vi "万能日期时间字符串解析.vi"(6 "分隔符(空格)":string=" " caption="日期时间分隔符(空格)", 11 "日期时间字符串":string="2017/12.30 12-12_12") -> (3 "时间标识":timestamp, 4 "格式":enum16{"无意义", "日期时间", "仅日期", "仅时间"}(ring))   [LabVIEW 2017]
uses:
  <vilib>/Utility/miscctls.llb/LVDateTimeRec.ctl
panel:
  out "6":string
  out "5":string
  out "4":string
  out "3":string
  out "2":string
  out "1":string
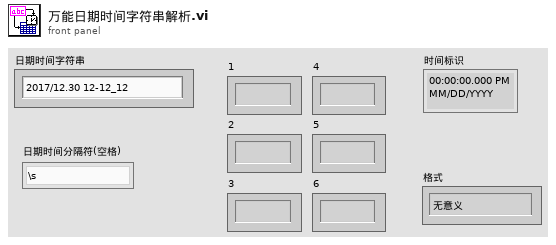
[diagram p1: front panel]
types:
  T1 = typedef "LVDateTimeRec.ctl" = cluster{"fractional second":dbl, "second":i32, "minute":i32, "hour":i32, "day of month":i32, "month":i32, "year":i32, "day of week":i32, "day of year":i32, "DST":i32}
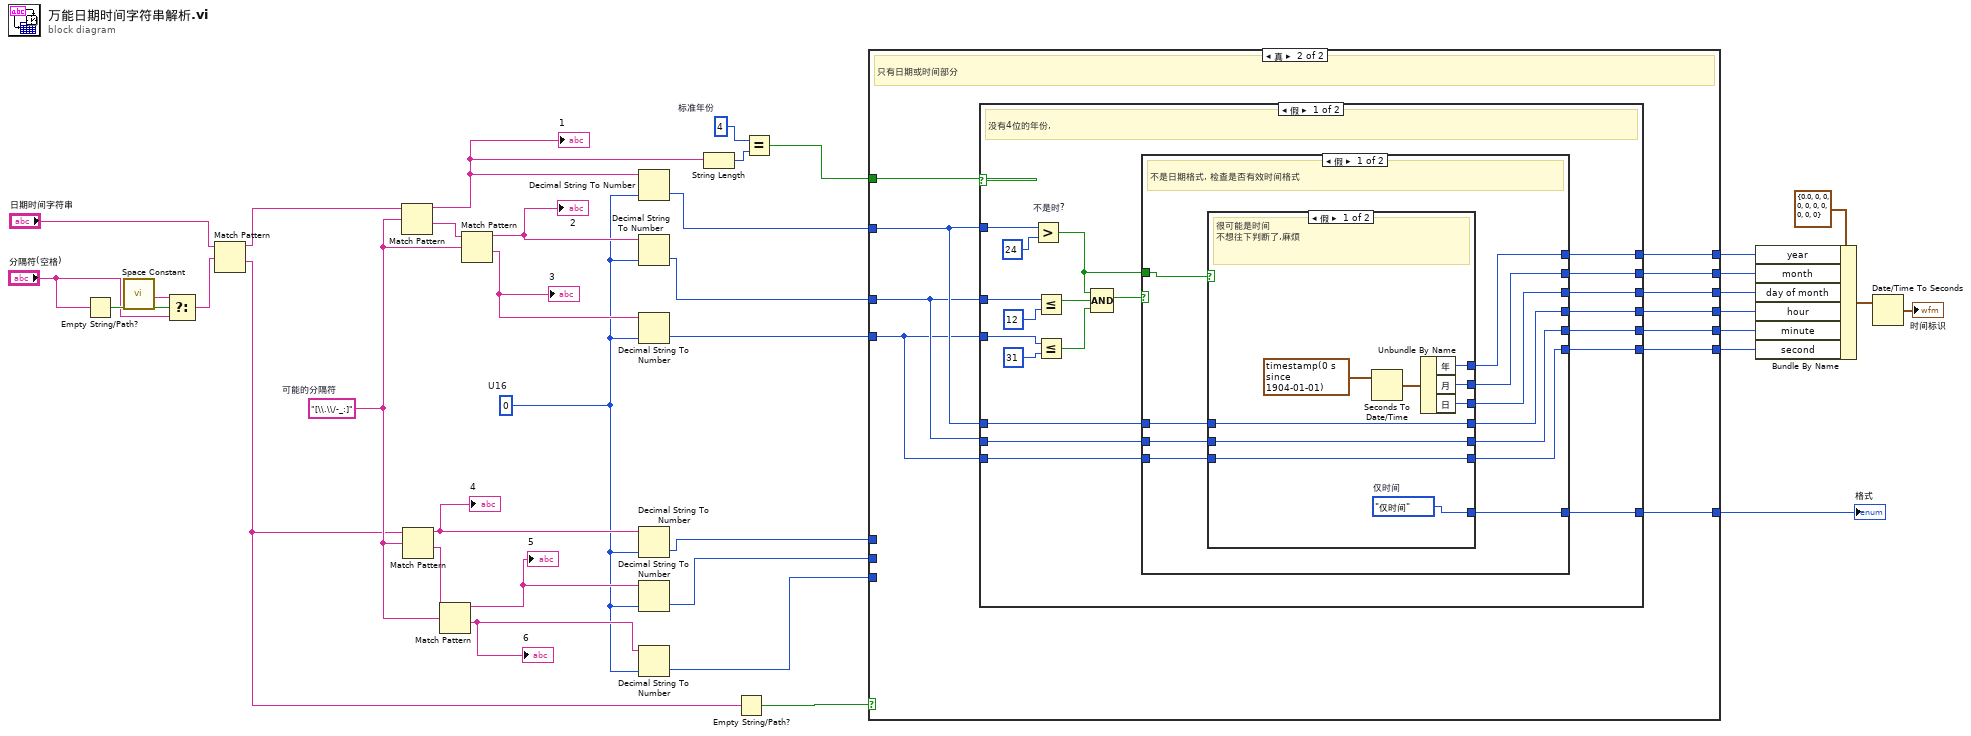
[diagram p0: block diagram]
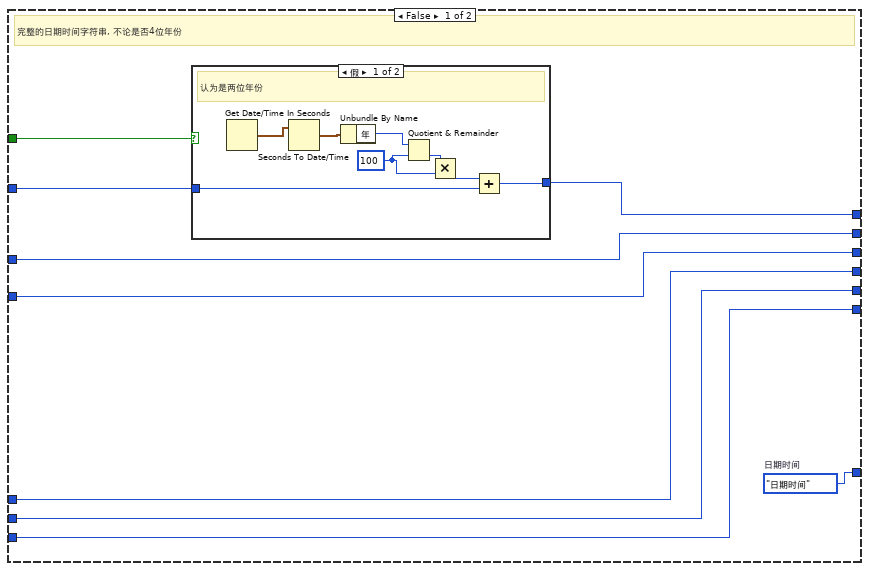
[diagram p2: hidden frame]
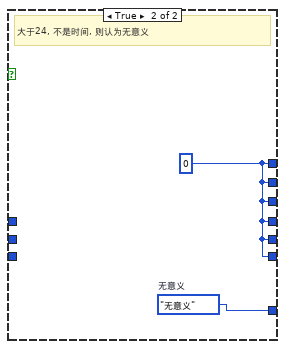
[diagram p4: hidden frame]
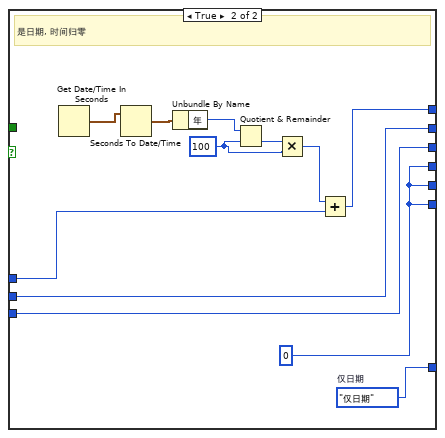
[diagram p5: hidden frame]
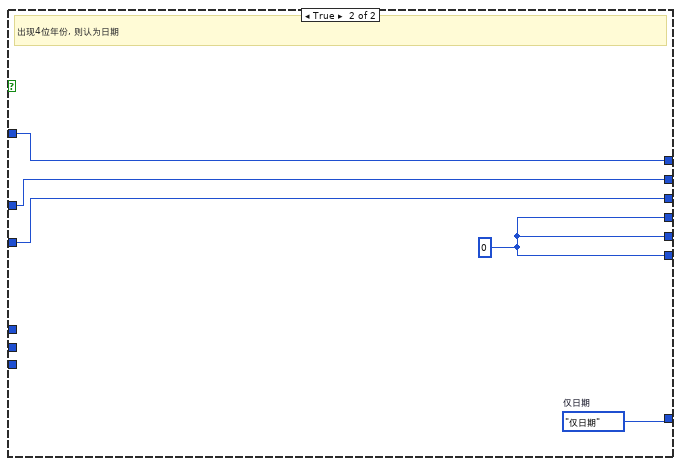
[diagram p6: hidden frame]
diagram:
  w22 = u16 0  # U16
  w24 = 4  # 标准年份
  w34 = "[\\.\\/-_:]"  # 可能的分隔符
  n1 = Empty String/Path?(string/path="分隔符(空格)") -> (empty?=w4:bool)
  n2 = call <vilib>:"Space Constant.vi"() -> ("String"=w3:string)
  n3 = Select(t=w3, s=w4, f="分隔符(空格)") -> (s? t:f=w1:string)
  n4 = Match Pattern(string="日期时间字符串", regular expression=w1) -> (before substring=w36:string, after substring=w27:string)  [unwired: 1 in, 2 out]
  n5 = Match Pattern(string=w36, regular expression=w34) -> (before substring=w26:string, after substring=w35:string)  [unwired: 1 in, 2 out]
  "1" <- w26
  n6 = Match Pattern(string=w27, regular expression=w34) -> (before substring=w30:string, after substring=w33:string)  [unwired: 1 in, 2 out]
  "4" <- w30
  n7 = Match Pattern(string=w33, regular expression=w34) -> (before substring=w29:string, after substring=w28:string)  [unwired: 1 in, 2 out]
  "5" <- w29
  "6" <- w28
  n8 = Match Pattern(string=w35, regular expression=w34) -> (before substring=w32:string, after substring=w31:string)  [unwired: 1 in, 2 out]
  "2" <- w32
  "3" <- w31
  n9 = Decimal String To Number(string=w26, default (0L)=w22) -> (number=w20:u16)  [unwired: 1 in, 1 out]
  n10 = Decimal String To Number(string=w32, default (0L)=w22) -> (number=w19:u16)  [unwired: 1 in, 1 out]
  n11 = Decimal String To Number(string=w31, default (0L)=w22) -> (number=w18:u16)  [unwired: 1 in, 1 out]
  n12 = Decimal String To Number(string=w30, default (0L)=w22) -> (number=w17:u16)  [unwired: 1 in, 1 out]
  n13 = Decimal String To Number(string=w29, default (0L)=w22) -> (number=w16:u16)  [unwired: 1 in, 1 out]
  n14 = Decimal String To Number(string=w28, default (0L)=w22) -> (number=w15:u16)  [unwired: 1 in, 1 out]
  n15 = String Length(string=w26) -> (length=w25:i32)
  n16 = Empty String/Path?(string/path=w27) -> (empty?=w23:bool)
  n17 = Equal?(x=w24, y=w25) -> (x = y?=w21:bool)
  n18 = case shown="真" w23 {
    tunnel: w21 -> [w46 w66]
    tunnel: w20 -> [w45 w59]
    tunnel: w19 -> [w43 w58]
    tunnel: w18 -> [w42 w57]
    tunnel: w17 -> [w41 _]
    tunnel: w16 -> [w40 _]
    tunnel: w15 -> [w39 _]
    tunnel: [w44 w65] -> w12
    tunnel: [w43 w64] -> w11
    tunnel: [w42 w63] -> w10
    tunnel: [w41 w62] -> w9
    tunnel: [w40 w61] -> w8
    tunnel: [w39 w60] -> w7
    tunnel: [w38 w56] -> w5
    frame False {
      w38 = enum16{"无意义", "日期时间", "仅日期", "仅时间"}."日期时间"  # 日期时间
      # "完整的日期时间字符串, 不论是否4位年份"
      n19 = case shown="假" w46 {
        tunnel: w45 -> [w50 w55]
        tunnel: [w49 w55] -> w44
        frame False {
          w47 = 100 ("y")
          # "认为是两位年份"
          n20 = Get Date/Time In Seconds() -> (seconds since 1Jan1904=w54:timestamp)
          n21 = Seconds To Date/Time(time stamp (now)=w54) -> (date time rec=w53:T1)  [unwired: 1 in]
          n22 = Unbundle By Name(w53) -> ("年"=w52:i32)
          n23 = Quotient & Remainder(x=w52, y=w47) -> (floor(x/y)=w51:i32)  [unwired: 1 out]
          n24 = Multiply(x=w51, y=w47) -> (x*y=w48:i32)
          n25 = Add(x=w48, y=w50) -> (x+y=w49:i32)
        }
        frame True {
          # "4位年份"
        }
      }
    }
    frame True {
      # "只有日期或时间部分"
      n26 = case shown="假" w66 {
        tunnel: w59 -> [w86 w125]
        tunnel: w58 -> [w84 w124]
        tunnel: w57 -> [w82 w123]
        tunnel: [w76 w125] -> w65
        tunnel: [w75 w124] -> w64
        tunnel: [w74 w123] -> w63
        tunnel: [w70 w122] -> w62
        tunnel: [w69 w122] -> w61
        tunnel: [w68 w122] -> w60
        tunnel: w59 -> [w73 _]
        tunnel: w58 -> [w72 _]
        tunnel: w57 -> [w71 _]
        tunnel: [w67 w121] -> w56
        frame False {
          # "没有4位的年份,"
          n27 = Greater? "不是时?"(x=w86, y=u16 24) -> (0:w77:bool)
          n28 = Less Or Equal?(x=w84, y=u16 12) -> (x <= y?=w79:bool)
          n29 = Less Or Equal?(x=w82, y=u16 31) -> (x <= y?=w78:bool)
          n30 = Compound Arithmetic op=AND ("复合运算")(w77, w79, w78) -> (w80:bool)
          n31 = case shown="假" w80 {
            tunnel: w77 -> [w97 _]
            tunnel: [w96 w112] -> w76
            tunnel: [w95 w120] -> w75
            tunnel: [w94 w119] -> w74
            tunnel: w73 -> [w93 w113]
            tunnel: w72 -> [w92 w120]
            tunnel: w71 -> [w91 w119]
            tunnel: [w90 w118] -> w70
            tunnel: [w89 w118] -> w69
            tunnel: [w88 w118] -> w68
            tunnel: [w87 w109] -> w67
            frame False {
              # "不是日期格式, 检查是否有效时间格式"
              n32 = case shown="假" w97 {
                tunnel: [w104 w108] -> w96
                tunnel: [w103 w108] -> w95
                tunnel: [w102 w108] -> w94
                tunnel: w93 -> [w101 _]
                tunnel: w92 -> [w100 _]
                tunnel: w91 -> [w99 _]
                tunnel: [w101 w108] -> w90
                tunnel: [w100 w108] -> w89
                tunnel: [w99 w108] -> w88
                tunnel: [w98 w107] -> w87
                frame False {
                  w98 = enum16{"无意义", "日期时间", "仅日期", "仅时间"}."仅时间"  # 仅时间
                  # "很可能是时间\n不想往下判断了,麻烦"
                  n33 = Seconds To Date/Time(time stamp (now)=timestamp(0 s since 1904-01-01) ("时间标识")) -> (date time rec=w106:T1)  [unwired: 1 in]
                  n34 = Unbundle By Name(w106) -> ("年"=w104:i32, "月"=w103:i32, "日"=w102:i32)
                }
                frame True {
                  w107 = enum16{"无意义", "日期时间", "仅日期", "仅时间"}."无意义"  # 无意义
                  w108 = 0 ("年")
                  # "大于24, 不是时间, 则认为无意义"
                }
              }
            }
            frame True {
              w109 = enum16{"无意义", "日期时间", "仅日期", "仅时间"}."仅日期"  # 仅日期
              w110 = 100 ("y")
              w118 = 0 ("年")
              # "是日期, 时间归零"
              n35 = Get Date/Time In Seconds() -> (seconds since 1Jan1904=w117:timestamp)
              n36 = Seconds To Date/Time(time stamp (now)=w117) -> (date time rec=w116:T1)  [unwired: 1 in]
              n37 = Unbundle By Name(w116) -> ("年"=w115:i32)
              n38 = Quotient & Remainder(x=w115, y=w110) -> (floor(x/y)=w114:i32)  [unwired: 1 out]
              n39 = Multiply(x=w114, y=w110) -> (x*y=w111:i32)
              n40 = Add(x=w111, y=w113) -> (x+y=w112:i32)
            }
          }
        }
        frame True {
          w121 = enum16{"无意义", "日期时间", "仅日期", "仅时间"}."仅日期"  # 仅日期
          w122 = u16 0 ("数字")
          # "出现4位年份, 则认为日期"
        }
      }
    }
  }
  "格式" <- w5
  n41 = Bundle By Name(cluster=T1 {"fractional second"=0.0, "second"=0, "minute"=0, "hour"=0, "day of month"=0, "month"=0, "year"=0, "day of week"=0, "day of year"=0, "DST"=0} ("日期时间记录"), "year"=w12, "month"=w11, "day of month"=w10, "hour"=w9, "minute"=w8, "second"=w7) -> (w14:T1)
  n42 = Date/Time To Seconds(2:w14) -> (0:→"时间标识":timestamp)  [unwired: 1 in]
